vi "Create Object.vi"(11 "jettl Queue Actor in":refnum<class "jettl Queue Actor.lvclass">) -> (2 "jettl Queue Actor":refnum<class "jettl Queue Actor.lvclass">)   [LabVIEW 2021, in "jettl.lvlib" / "jettl Queue Actor.lvlib" / "jettl Queue Actor.lvclass"]
uses:
  jettl Queue Actor.lvclass
  jettl.lvlib
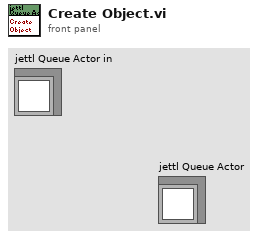
[diagram p1: front panel]
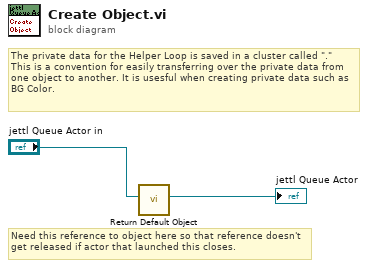
[diagram p0: block diagram]
diagram:
  # "The private data for the Helper Loop is saved in a cluster called \".\"\nThis is a convention for easily transferring over the private data from one object to another. It is usesful when creating private data such as BG Color."
  # "Need this reference to object here so that reference doesn't get released if actor that launched this closes."
  n1 = call "Return Default Object.vi"("Object"="jettl Queue Actor in") -> ("Default Object Instance"=→"jettl Queue Actor":refnum<class "jettl Queue Actor.lvclass">)  [unwired: 10 in]
